vi "PH_PLH-AccessInformation.get i attribute.vi"(0 "i ref in":refnum<vi>, 5 "error in (no error)":errorcluster) -> (14 "i ref out":refnum<vi>, 16 "i attribute":T1 {"Searchmode" items=["Searchmode: no info", "no Searchmode", "Searchmode"]; "Shotmode" items=["Shotmode: no info", "no Shotmode", "Shotmode"]}, 19 "error out":errorcluster)   [LabVIEW 2014, in "PH_PLH-AccessInformation.lvlib"]
doc: "Gets the i attribute data of an object.\n\nLicense Agreement for this software:\n\nCopyright (C)\nGesellschaft für Schwerionenforschung, GSI\nPlanckstr. 1\n64291 Darmstadt\nGermany\n\nContact: D.Beck@gsi.de \n\nThis program is free software; you can redistribute it and/or modify it under the terms of the GNU General Public License as published by the Free Software Foundation; either version 2 of the license, or (at your option) any later version.\n\nThis program is distributed in the hope that it will be useful, but WITHOUT ANY WARRANTY; without even the implied warranty of MERCHANTABILITY or FITNESS FOR A PARTICULAR PURPOSE. See the GNU General License for more details (http://www.gnu.org).\n\nGesellschaft für Schwerionenforschung, GSI\nPlanckstr. 1, 64291 Darmstadt, Germany\nFor all questions and ideas contact: M.Richter@gsi.de, H.Brand@gsi.de or D.Beck@gsi.de.\nLast update: 17-JUN-2004"
uses:
  PH_PLH-AccessInformation.lvlib
  PH_PLH-AccessInformation.i attribute.ctl
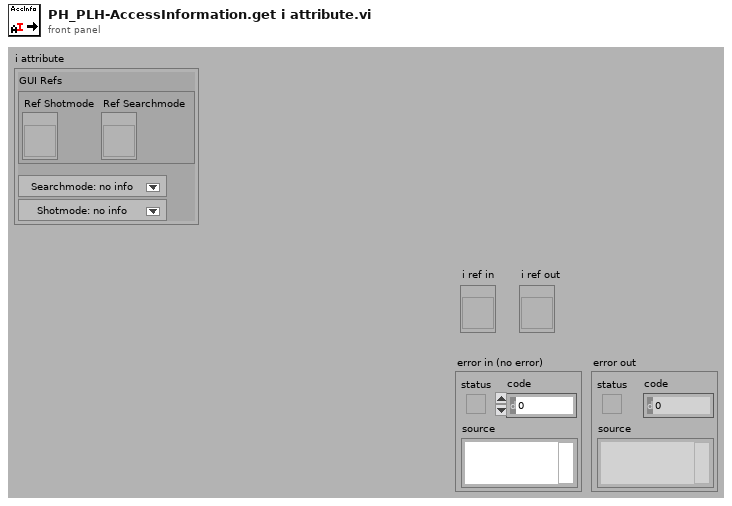
[diagram p1: front panel]
types:
  T1 = typedef "PH_PLH-AccessInformation.lvlib/PH_PLH-AccessInformation.i attribute.ctl" = cluster{"GUI Refs":cluster{"Ref Shotmode":refnum<vi>, "Ref Searchmode":refnum<vi>}, "Shotmode":i32, "Searchmode":i32}
  T2 = enum16{"SetAttribute", "GetAttribute", "CreateAttribute", "DestroyAttribute", "DestroyAllAtributes"}
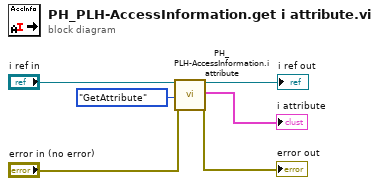
[diagram p0: block diagram]
diagram:
  n1 = call "PH_PLH-AccessInformation.i attribute.vi"("VI Refnum"="i ref in", "Action"=T2."GetAttribute", "error in (no error)"="error in (no error)") -> ("VI Refnum out"=→"i ref out":refnum<vi>, "CLASS.i attribute out"=→"i attribute":T1, "error out"=→"error out":errorcluster)  [unwired: 14 in]
